vi "Msg To Caller.vi"(9 "Priority?":bool, 10 "Msg":refnum<class "Msg.lvclass">, 11 "jettl Queue Actor in":refnum<class "jettl Queue Actor.lvclass">) -> (0 "error out":errorcluster)   [LabVIEW 2021, in "jettl.lvlib" / "jettl Queue Actor.lvlib" / "jettl Queue Actor.lvclass"]
uses:
  jettl Queue Actor.lvclass
  Actor/Msg/Msg.lvclass
  jettl Queue Actor.lvclass/jettl Queue Actor.ctl
  jettl.lvlib
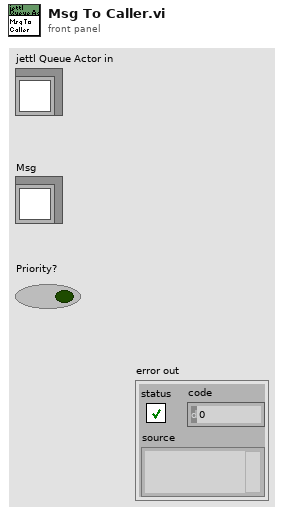
[diagram p1: front panel]
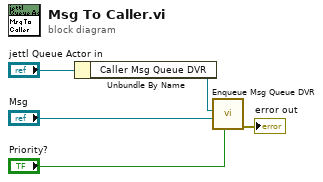
[diagram p0: block diagram]
diagram:
  n1 = Unbundle By Name("jettl Queue Actor in") -> ("Caller Msg Queue DVR"=w5:refnum<data-value>)
  n2 = call "Enqueue Msg Queue DVR.vi"("Priority?"="Priority?", "Msg"="Msg", "Msg Queue DVR"=w5) -> ("error out"=→"error out":errorcluster)  [unwired: 8 in]
